vi "Busy Timeout.vi"(8 "error in (no error)":errorcluster, 10 "busy timeout (ms)":i32=5000, 11 "Connection in":refnum<class "Connection.lvclass">) -> (0 "error out":errorcluster, 3 "Connection out":refnum<class "Connection.lvclass">)   [LabVIEW 2023, in "SQLiteSupport.lvlib" / "Connection.lvclass"]
doc: "Sets the Busy Timeout of the Connection: the time opertions such as \"Step\" will wait when the database is locked by another connection before returning an error."
uses:
  Connection.lvclass
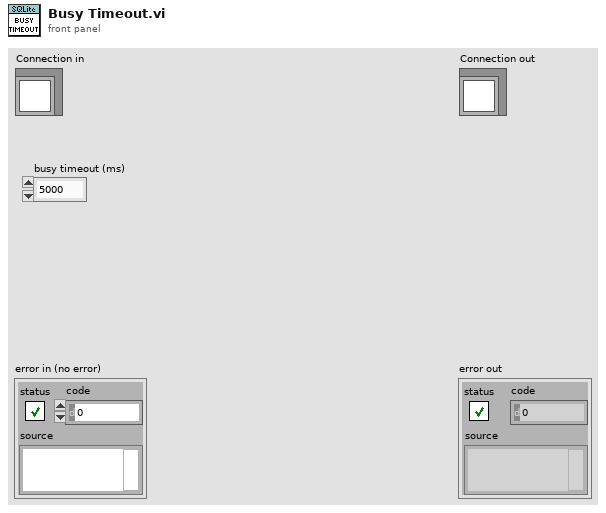
[diagram p1: front panel]
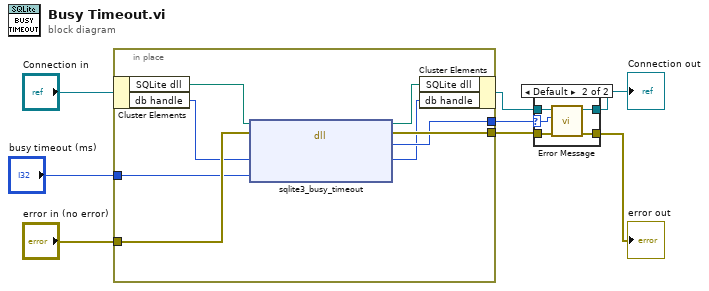
[diagram p0: block diagram]
diagram:
  n1 = in-place {
    in-place-border: "error in (no error)" -> [w16]
    in-place-border: "busy timeout (ms)" -> [w15]
    in-place-border: [w14] -> w6
    in-place-border: [w13] -> w5
    n2 = in-place-cluster #1("Connection in") -> ("SQLite dll"=w9:path, "db handle"=w12:u64)
    n3 = dll-call lib="C:/LabVIEW_JDP/Support/SQLite/SQL Connection/sqlite3.dll" fn="sqlite3_busy_timeout"(path in=w9, error in=w16, "handle"=w12, "timeout (ms)"=w15) -> (path out=w10:path, error out=w14:errorcluster, "return code"=w13:i32, "handle"=w11:u64)  [unwired: 2 in]
    n4 = in-place-cluster #1("SQLite dll"=w10, "db handle"=w11) -> (w2:refnum<class "Connection.lvclass">)
  }
  n5 = case shown="Default" w5 {
    selector: w5 -> [_ w20]
    tunnel: [w17 w23] -> w1
    tunnel: w6 -> [w18 w22]
    tunnel: [w18 w21] -> w4
    tunnel: w2 -> [w17 w19]
    frame 0 {
      # "No Error"
    }
    frame Default {
      n6 = call "Error Message.vi"("error in (no error)"=w22, "error code"=w20, "Connection in"=w19) -> ("error out"=w21:errorcluster, "Connection out"=w23:refnum<class "Connection.lvclass">)  [unwired: 7 in]
    }
  }
  "error out" <- w4
  "Connection out" <- w1
